vi "LINSERT.vi"(0 "refnum in":refnum<vi>, 1 "Key":string, 2 "Order":enum16{"BEFORE", "AFTER"}(ring), 5 "Pivot":string, 7 "Value":string, 11 "error in":errorcluster) -> (4 "refnum out":refnum<vi>, 6 "Data":T1, 15 "error out":errorcluster)   [LabVIEW 2023]
uses:
  SubVIs/Controls/redis-data.ctl
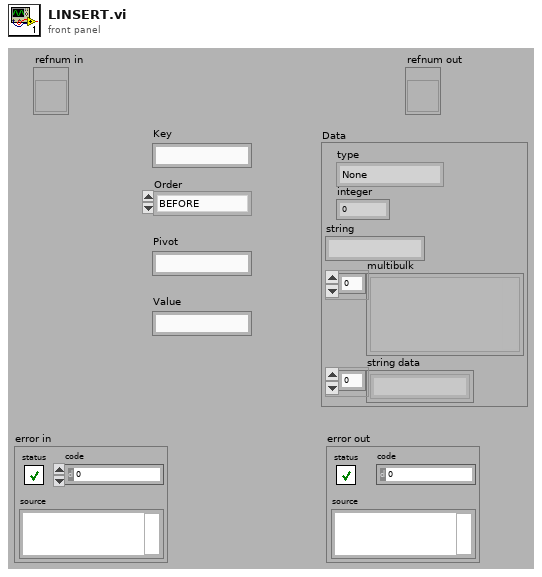
[diagram p1: front panel]
types:
  T1 = typedef "redis-data.ctl" = cluster{"type":enum16{"None", "Error", "Status", "Nil", "Integer", "String", "Multibulk"}, "integer":i64, "string":string, "multibulk":variant[], "string data":string[]}
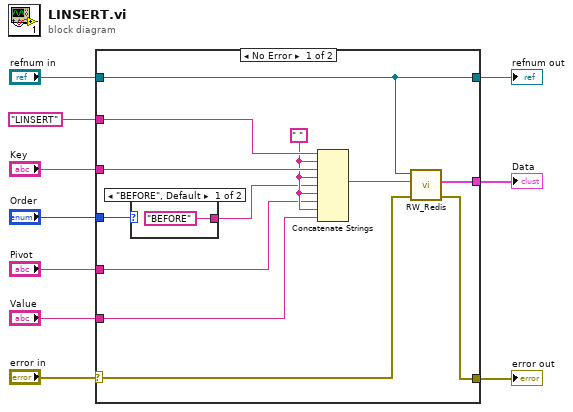
[diagram p0: block diagram]
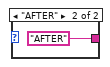
[diagram p2: hidden frame]
diagram:
  n1 = case shown="No Error" "error in" {
    selector: "error in" -> [w21 w26]
    tunnel: "Key" -> [w18 _]
    tunnel: "LINSERT" -> [w22 _]
    tunnel: "refnum in" -> [w17 w25]
    tunnel: [w20 w26] -> w8
    tunnel: [w19 _] -> w4
    tunnel: [w17 w25] -> w6
    tunnel: "Order" -> [w16 _]
    tunnel: "Pivot" -> [w13 _]
    tunnel: "Value" -> [w12 _]
    frame No Error {
      w15 = " "
      n2 = case shown="\"BEFORE\", Default" w16 {
        tunnel: ["BEFORE" "AFTER"] -> w14
        frame "BEFORE", Default {
        }
        frame "AFTER" {
        }
      }
      n3 = Concatenate Strings(w22, w15, w18, w15, w14, w15, w13, w15, w12) -> (w11:string)
      n4 = call "RW_Redis.vi"("error in"=w21, "command"=w11, "refnum"=w17) -> ("error out"=w20:errorcluster, "Data"=w19:T1)  [unwired: 7 in]
    }
    frame Error {
    }
  }
  "error out" <- w8
  "Data" <- w4
  "refnum out" <- w6
